vi "Firma.vi"() -> ()   [LabVIEW 2017]
uses:
  <vilib>/Utility/miscctls.llb/LVMouseTypeDef.ctl
panel:
  out "Boolean 2":bool=TRUE
  out "Boolean":bool=TRUE
  out "size(s) 2":i32
  out "size(s)":i32
  in  "file path (use dialog) 2":path=path "C:/Users/LuisFernando/Documents/UPIITA/8vo semestre/Instrumentacion Virtual Aplicada/Solidworks/Sistema_Coordenado_Lectura/Archivos_Lectura/EjeY.txt"
  in  "file path (use dialog)":path=path "C:/Users/LuisFernando/Documents/UPIITA/8vo semestre/Instrumentacion Virtual Aplicada/Solidworks/Sistema_Coordenado_Lectura/Archivos_Lectura/EjeX.txt"
  out "XY Graph":cluster{i32[], i32[]}(graph)
  out "Waveform Graph 2":i32[](graph)
  out "Waveform Graph":i32[](graph)
  out "Mouse":T1
  in  "Stop Button":bool
  out "2D Picture":picture
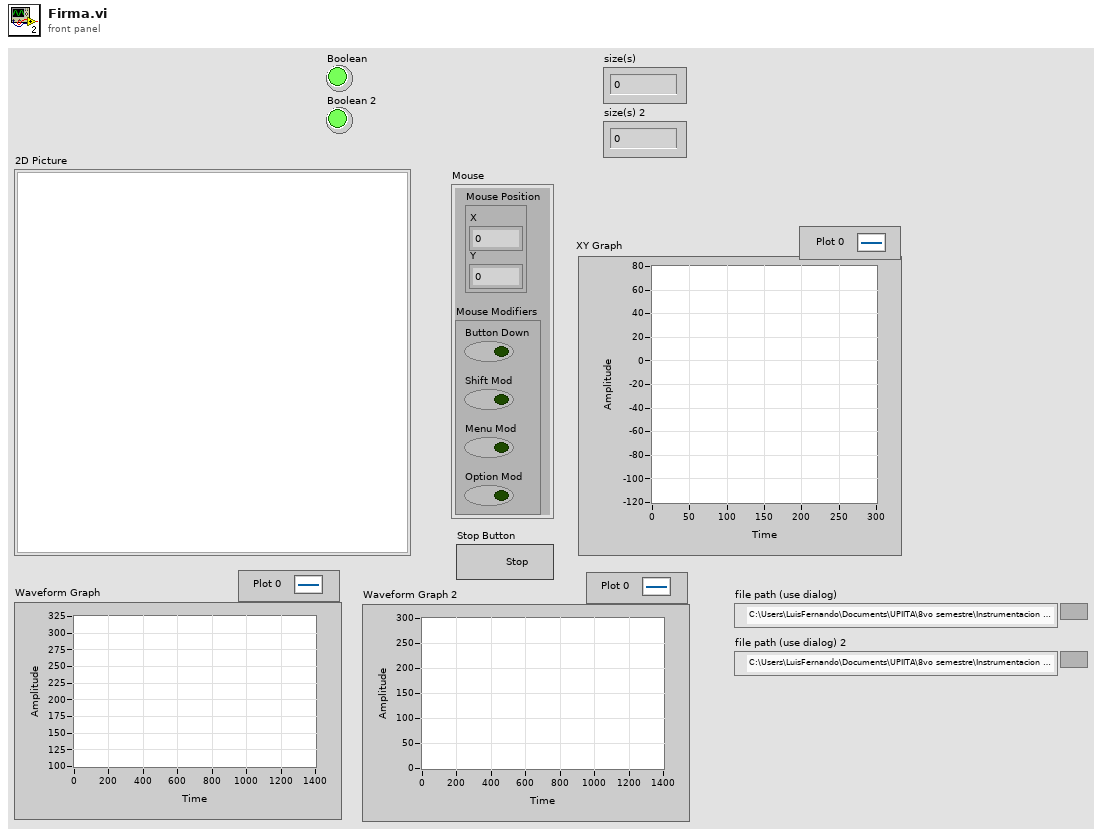
[diagram p1: front panel]
types:
  T1 = typedef "LVMouseTypeDef.ctl" = cluster{"Mouse Position":cluster{"X":i32, "Y":i32}, "Mouse Modifiers":cluster{"Button Down":bool, "Shift Mod":bool, "Menu Mod":bool, "Option Mod":bool}}
  T2 = enum16{"open", "replace", "create", "open or create", "replace or create", "replace or create with confirmation"}
  T3 = cluster{"Width":u16, "Style":enum32{"Solid", "Dash", "Dot", "DashDot", "DashDotDot"}}
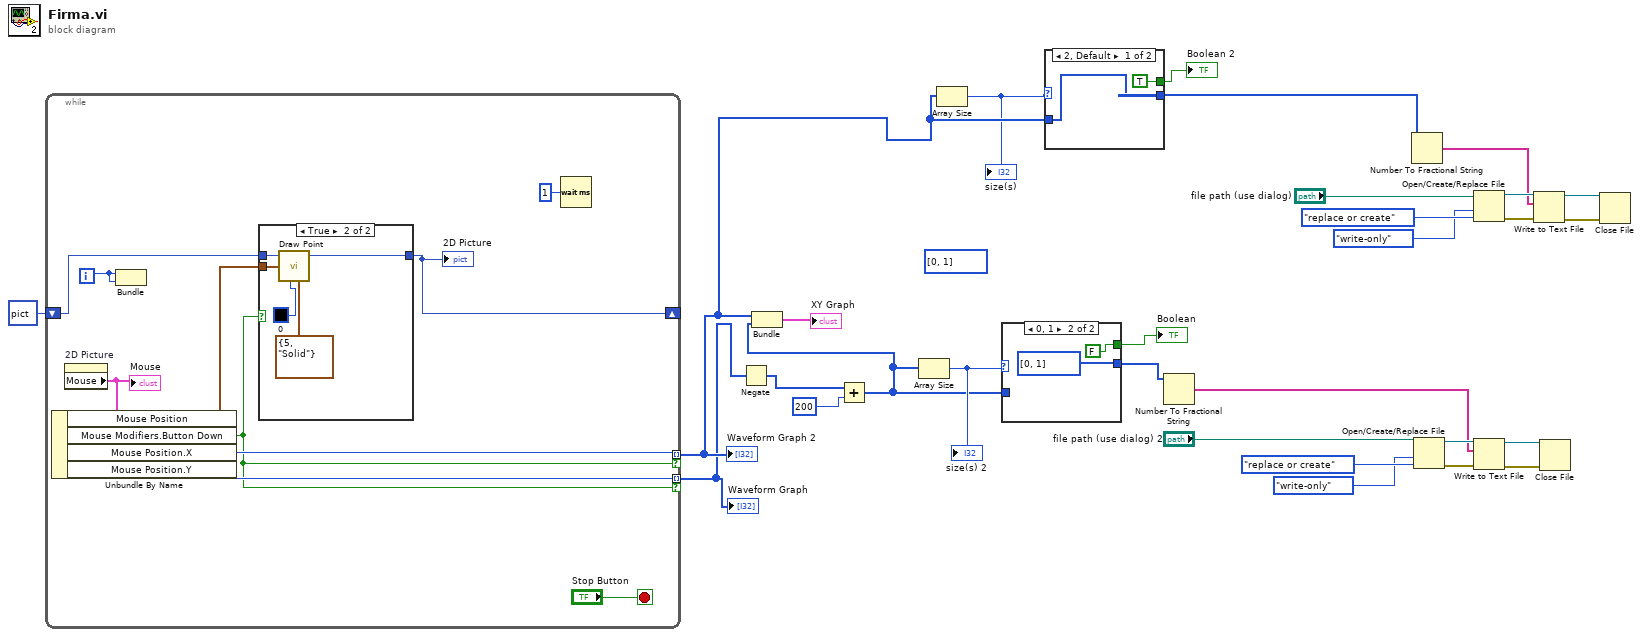
[diagram p0: block diagram]
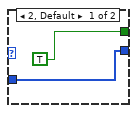
[diagram p2: hidden frame]
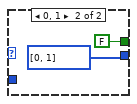
[diagram p3: hidden frame]
diagram:
  (unwired) i32[] [0, 1] ("Array")
  n1 = while {
    shift-right: [w37] -> _
    shift-left: picture data[5B] ("new picture") -> [w36]
    tunnel: [w32] -> w9 mode=indexing if=w30
    tunnel: [w31] -> w6 mode=indexing if=w30
    i -> [w39]
    stop <- "Stop Button" stop-if-true
    n2 = property on="2D Picture" class="Pict"() -> ("Mouse"=w34:T1)  [unwired: 2 in, 2 out]
    "Mouse" <- w34
    n3 = Unbundle By Name(w34) -> ("Mouse Position"=w33:cluster{"X":i32, "Y":i32}, "Mouse Modifiers.Button Down"=w30:bool, "Mouse Position.X"=w32:i32, "Mouse Position.Y"=w31:i32)
    n4 = Bundle(w39, w39) -> ()  [unwired: 1 in, 1 out]
    n5 = case shown="True" w30 {
      tunnel: [w40 w44] -> w37
      tunnel: w36 -> [w40 w43]
      tunnel: w33 -> [_ w42]
      frame False {
      }
      frame True {
        n6 = call <vilib>:"Draw Point.vi"("picture"=w43, "point(x,y)"=w42, "color(black)"=u32 0, "pen"=T3 {"Width"=5, "Style"=enum."Solid"}) -> ("new picture"=w44:picture)  [unwired: 5 in]
      }
    }
    "2D Picture" <- w37
    n7 = Wait (ms)(milliseconds to wait=u32 1) -> ()  [unwired: 1 out]
  }
  "Waveform Graph" <- w6
  "Waveform Graph 2" <- w9
  n8 = Negate(x=w6) -> (-x=w8:i32[])
  n9 = Add(x=w8, y=200) -> (x+y=w5:i32[])
  n10 = Bundle(w9, w5) -> (→"XY Graph":cluster{i32[], i32[]})  [unwired: 1 in]
  n11 = Array Size(array=w5) -> (size(s)=w26:i32)
  "size(s) 2" <- w26
  n12 = Array Size(array=w9) -> (size(s)=w4:i32)
  "size(s)" <- w4
  n13 = case shown="0, 1" w26 {
    tunnel: w5 -> [w47 _]
    tunnel: [w47 i32[] [0, 1] ("Array")] -> w3
    tunnel: [TRUE ("Boolean") FALSE ("Boolean")] -> w2
    frame 2, Default {
    }
    frame 0, 1 {
    }
  }
  "Boolean" <- w2
  n14 = case shown="2, Default" w4 {
    tunnel: [w51 i32[] [0, 1] ("Array")] -> w27
    tunnel: w9 -> [w51 _]
    tunnel: [TRUE ("Boolean") FALSE ("Boolean")] -> w1
    frame 2, Default {
    }
    frame 0, 1 {
    }
  }
  "Boolean 2" <- w1
  n15 = Number To Fractional String(number=w3) -> (F-format string=w10:string[])  [unwired: 3 in]
  n16 = Number To Fractional String(number=w27) -> (F-format string=w18:string[])  [unwired: 3 in]
  n17 = Open/Create/Replace File(file path (use dialog)="file path (use dialog) 2", operation (0:open)=T2."replace or create", access (0:read/write)=enum16{"read/write", "read-only", "write-only"}."write-only") -> (refnum out=w17:refnum<file>, error out=w16:errorcluster)  [unwired: 3 in, 1 out]
  n18 = Open/Create/Replace File(file path (use dialog)="file path (use dialog)", operation (0:open)=T2."replace or create", access (0:read/write)=enum16{"read/write", "read-only", "write-only"}."write-only") -> (refnum out=w25:refnum<file>, error out=w24:errorcluster)  [unwired: 3 in, 1 out]
  n19 = Write to Text File(file (use dialog)=w17, text=w10, error in=w16) -> (refnum out=w15:refnum<file>, error out=w14:errorcluster)  [unwired: 1 in, 1 out]
  n20 = Write to Text File(file (use dialog)=w25, text=w18, error in=w24) -> (refnum out=w23:refnum<file>, error out=w22:errorcluster)  [unwired: 1 in, 1 out]
  n21 = Close File(refnum=w15, error in=w14) -> ()  [unwired: 2 out]
  n22 = Close File(refnum=w23, error in=w22) -> ()  [unwired: 2 out]
